vi "PRIME Telescope Converstion test program.vi"() -> ()   [LabVIEW 2024, in "PRIME Telescope.lvclass"]
uses:
  PRIME Telescope.lvclass
panel:
  out "Dec String 2":string
  out "RA String 2":string
  out "output cluster 2":cluster{"RA":dbl, "DEC":dbl}
  out "output cluster":cluster{"RA":dbl, "DEC":dbl}
  in  "Dec String":string
  in  "RA String":string
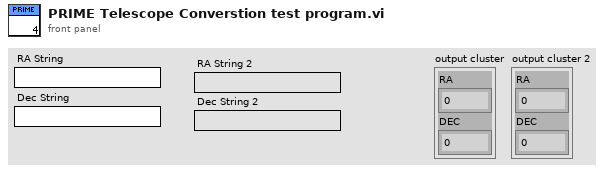
[diagram p1: front panel]
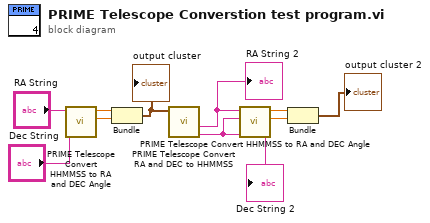
[diagram p0: block diagram]
diagram:
  n1 = call "PRIME Telescope Convert HHMMSS to RA and DEC Angle.vi"("Dec String"="Dec String", "RA String"="RA String") -> ("DEC"=w7:dbl, "RA"=w8:dbl)  [unwired: 7 in, 1 out]
  n2 = Bundle("RA"=w8, "DEC"=w7) -> (w6:cluster{"RA":dbl, "DEC":dbl})  [unwired: 1 in]
  "output cluster" <- w6
  n3 = call "PRIME Telescope Convert RA and DEC to HHMMSS.vi"("RA and DEC"=w6) -> ("Dec String"=w4:string, "RA String"=w5:string)  [unwired: 7 in, 2 out]
  "RA String 2" <- w5
  "Dec String 2" <- w4
  n4 = call "PRIME Telescope Convert HHMMSS to RA and DEC Angle.vi"("Dec String"=w4, "RA String"=w5) -> ("DEC"=w2:dbl, "RA"=w3:dbl)  [unwired: 7 in, 1 out]
  n5 = Bundle("RA"=w3, "DEC"=w2) -> (→"output cluster 2":cluster{"RA":dbl, "DEC":dbl})  [unwired: 1 in]
